vi "Symbol Value.vi"(11 "Open Symbol":T1) -> (3 "Corrupt Value":u64, 5 "Incomplete Val":u64)   [LabVIEW 2020]
uses:
  Open Symbol.ctl
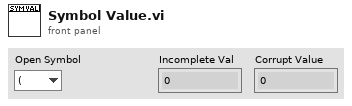
[diagram p1: front panel]
types:
  T1 = typedef "Open Symbol.ctl" = enum16{"(", "[", "{", "<"}
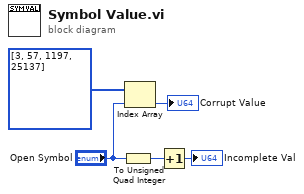
[diagram p0: block diagram]
diagram:
  n1 = To Unsigned Quad Integer(1:"Open Symbol") -> (0:w2:u64)
  n2 = Index Array(array=u64[] [3, 57, 1197, 25137], index="Open Symbol") -> (element=→"Corrupt Value":u64)
  n3 = Increment(x=w2) -> (x+1=→"Incomplete Val":u64)
